vi "MGI Print Image.vi"(8 "error in (no error)":errorcluster, 10 "Page Orientation":T1(ring)=enum."Landscape", 11 "image data":T2) -> (0 "error out":errorcluster)   [LabVIEW 2020]
doc: "Prints the specified image by drawing the image to the front panel's picture control and then printing the panel.\n\nAuthored by Shawn D. Walpole\nsupport@mooregoodideas.com\nwww.mooregoodideas.com\n\nCopyright (c) 2010, Moore Good Ideas, Inc.\n\nAll rights reserved.\n\nRedistribution and use in source and binary forms, with or without modification, are permitted provided that the following conditions are met:\n\n * Redistributions of source code must retain the above copyright notice, this list of conditions and the following disclaimer.\n * Redistributions in binary form must reproduce the above copyright notice, this list of conditions and the following disclaimer in the documentation and/or other materials provided with the distribution.\n * Neither the name of Moore Good Ideas, Inc. nor the names of its contributors may be used to endorse or promote products derived from this software without specific prior written permission.\n\nTHIS SOFTWARE IS PROVIDED BY THE COPYRIGHT HOLDERS AND CONTRIBUTORS \"AS IS\" AND ANY EXPRESS OR IMPLIED WARRANTIES, INCLUDING, BUT NOT LIMITED TO, THE IMPLIED WARRANTIES OF MERCHANTABILITY AND FITNESS FOR A PARTICULAR PURPOSE ARE DISCLAIMED. IN NO EVENT SHALL THE COPYRIGHT OWNER OR CONTRIBUTORS BE LIABLE FOR ANY DIRECT, INDIRECT, INCIDENTAL, SPECIAL, EXEMPLARY, OR CONSEQUENTIAL DAMAGES (INCLUDING, BUT NOT LIMITED TO, PROCUREMENT OF SUBSTITUTE GOODS OR SERVICES; LOSS OF USE, DATA, OR PROFITS; OR BUSINESS INTERRUPTION) HOWEVER CAUSED AND ON ANY THEORY OF LIABILITY, WHETHER IN CONTRACT, STRICT LIABILITY, OR TORT (INCLUDING NEGLIGENCE OR OTHERWISE) ARISING IN ANY WAY OUT OF THE USE OF THIS SOFTWARE, EVEN IF ADVISED OF THE POSSIBILITY OF SUCH DAMAGE."
uses:
  <vilib>/picture/picture.llb/imagedata.ctl
panel:
  out "Picture":picture
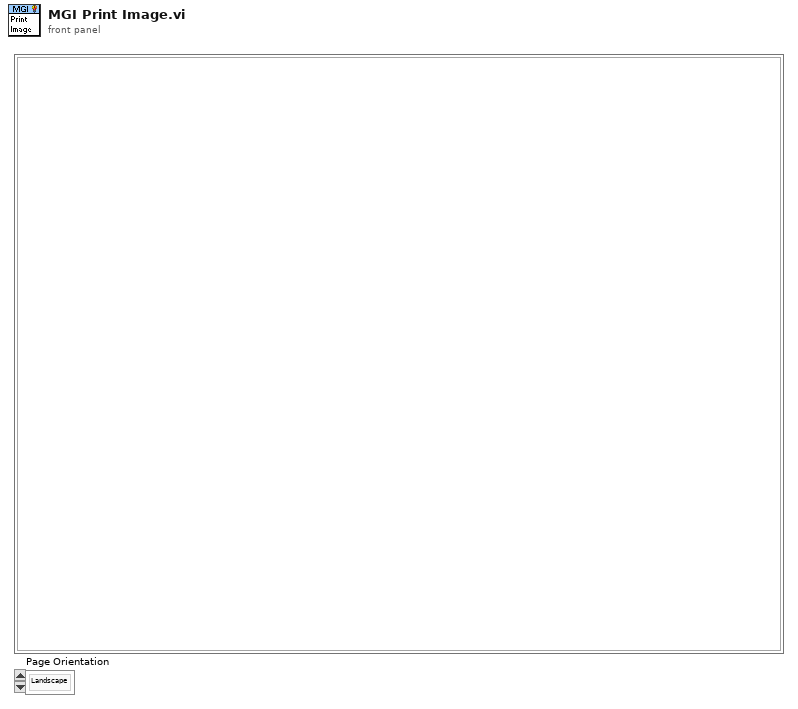
[diagram p1: front panel]
types:
  T1 = enum32{"Portrait", "Landscape", "Rotated Portrait", "Rotated Landscape"}
  T2 = typedef "imagedata.ctl" = cluster{"image type":i32, "image depth":i32, "image":u8[], "mask":u8[], "colors":u32[], "Rectangle":cluster{"left":i16, "top":i16, "right":i16, "bottom":i16}}
  T3 = cluster{"left":i16, "top":i16, "right":i16, "bottom":i16}
  T4 = typedef "LVBoundsTypeDef.ctl" = cluster{"Width":u32, "Height":u32}
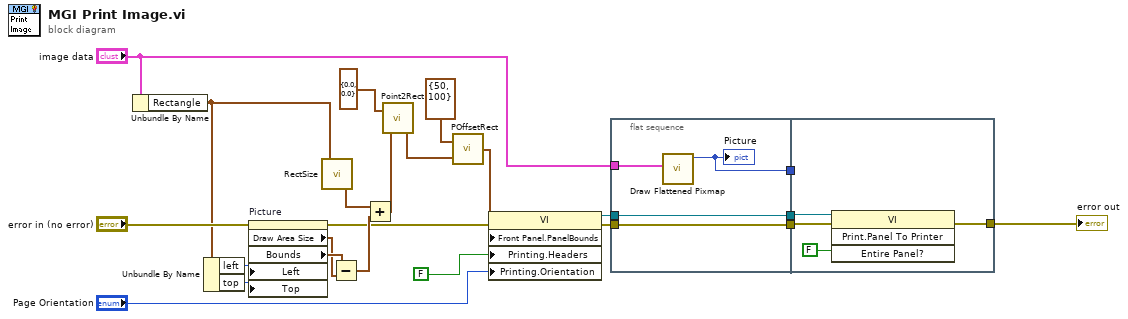
[diagram p0: block diagram]
diagram:
  n1 = Unbundle By Name("image data") -> ("Rectangle"=w8:T3)
  n2 = Unbundle By Name(w8) -> ("left"=w7:i16, "top"=w6:i16)
  n3 = property on="Picture" class="Pict"(error in="error in (no error)", "Left"=w7, "Top"=w6) -> (error out=w13:errorcluster, "Draw Area Size"=w15:T4, "Bounds"=w16:T4)  [unwired: 1 in, 1 out]
  n4 = call <vilib>:"RectSize.vi"("rect"=w8) -> ("point"=w12:cluster{"x":i16, "y":i16})
  n5 = Subtract(x=w16, y=w15) -> (x-y=w14:T4)
  n6 = Add(x=w12, y=w14) -> (x+y=w11:T4)
  n7 = call <vilib>:"Point2Rect.vi"("point b"=w11, "point a"=cluster{"x":dbl, "y":dbl} {"x"=0.0, "y"=0.0}) -> ("rect"=w21:T3)
  n8 = call <vilib>:"POffsetRect.vi"("rect"=w21, "point"=cluster{"x":i16, "y":i16} {"x"=50, "y"=100}) -> ("offset rect"=w20:T3)
  n9 = property class="VI"(error in=w13, "Front Panel.PanelBounds"=w20, "Printing.Headers"=FALSE ("Printing:Page Headers?"), "Printing.Orientation"="Page Orientation") -> (reference out=w19:refnum<vi>, error out=w18:errorcluster)  [unwired: 1 in]
  n10 = flat-sequence {
    tunnel: "image data" -> [w26]
    tunnel: w19 -> [w25]
    tunnel: w18 -> [w24]
    tunnel: [w27] -> w4
    tunnel: [w25] -> w3
    tunnel: [w24] -> w2
    tunnel: w4 -> [_]
    tunnel: w3 -> [w30]
    tunnel: w2 -> [w29]
    tunnel: [w28] -> w1
    frame #0 {
      n11 = call <vilib>:"Draw Flattened Pixmap.vi"("image data"=w26) -> ("new picture"=w27:picture)  [unwired: 1 in, 7 out]
      "Picture" <- w27
    }
    frame #1 {
      n12 = invoke class="VI" method="Print.Panel To Printer"(reference=w30, error in=w29, "Entire Panel?"=FALSE) -> (error out=w28:errorcluster)  [unwired: 1 in, 3 out]
    }
  }
  "error out" <- w1
